vi "Write Invert Inputs.vi"(5 "Invert Inputs":bool[](array[boolean]), 9 "CompoundArithmetic in":refnum<class "CompoundArithmetic.lvclass">) -> (3 "CompoundArithmetic out":refnum<class "CompoundArithmetic.lvclass">)   [LabVIEW 2014, in "CompoundArithmetic.lvclass"]
uses:
  CompoundArithmetic.lvclass
  CompoundArithmetic.lvclass/CompoundArithmetic.ctl
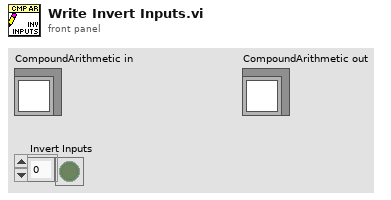
[diagram p1: front panel]
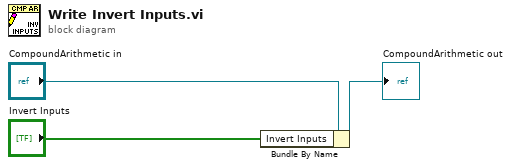
[diagram p0: block diagram]
diagram:
  n1 = Bundle By Name(cluster="CompoundArithmetic in", "Invert Inputs"="Invert Inputs") -> (→"CompoundArithmetic out":refnum<class "CompoundArithmetic.lvclass">)
